vi "写入password.vi"(8 "error in (no error)":errorcluster caption="错误输入（无错误）", 10 "password":string, 11 "database输入":refnum<class "database.lvclass">) -> (0 "error out":errorcluster caption="错误输出", 3 "database输出":refnum<class "database.lvclass">)   [LabVIEW 2016, in "中水三立SQL数据传输.lvlib" / "database.lvclass"]
uses:
  database.lvclass
  database.lvclass/database.ctl
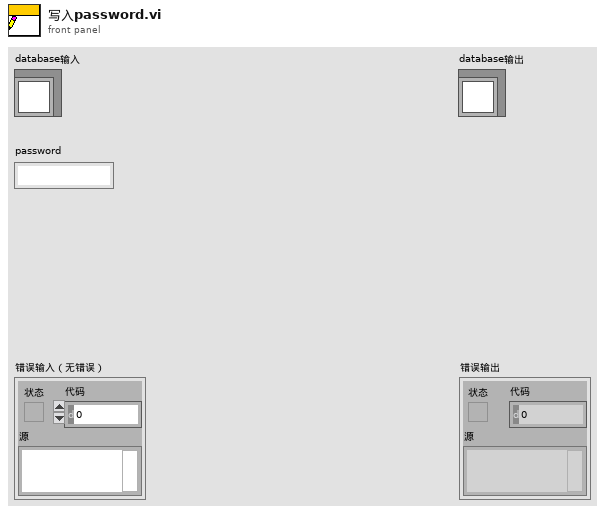
[diagram p1: front panel]
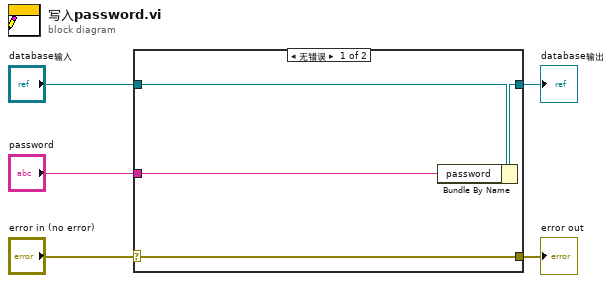
[diagram p0: block diagram]
diagram:
  n1 = case shown="无错误" "error in (no error)" {
    selector: "error in (no error)" -> [w9 w10]
    tunnel: [w9 w10] -> w4
    tunnel: [w7 w11] -> w2
    tunnel: "database输入" -> [w8 w11]
    tunnel: "password" -> [w6 _]
    frame No Error {
      n2 = Bundle By Name(cluster=w8, "password"=w6) -> (w7:refnum<class "database.lvclass">)
    }
    frame Error {
    }
  }
  "error out" <- w4
  "database输出" <- w2
